vi "G2CPU Complex Process.vi"(10 "Backend":T1 items=["Default Backend"=0, "CPU Backend"=1, "CUDA Backend"=2, "OPENCL Backend"=4, "Intel OneAPI"=8], 11 "X size":i32=16384) -> (3 "G2CPU Time":dbl)   [LabVIEW 2020]
uses:
  <vilib>/Natan Biesmans/G2CPU GPU and CPU HPC Toolkit/ArrayFire Driver/TypeDefs/backend.ctl
  fbbaf97c-3b5e-4b4c-bc14-40c3526c788b.vi
  c2200195-6f6b-46fb-afe8-d4cd0bcb91cf.vi
  fbbaf97c-3b5e-4b4c-bc14-40c3526c788b.vi/caaf1833-0905-411b-a9ed-2cc30d41907c.vi
  <vilib>/Natan Biesmans/G2CPU GPU and CPU HPC Toolkit/G2CPU Libraries/Arrays/SubVI/Array Sizes to Dim Cluster.vi
  c2200195-6f6b-46fb-afe8-d4cd0bcb91cf.vi/caaf1833-0905-411b-a9ed-2cc30d41907c.vi
  fbbaf97c-3b5e-4b4c-bc14-40c3526c788b.vi/caaf1833-0905-411b-a9ed-2cc30d41907c.vi/1a23f98f-393f-4176-8983-7f1ab824c539.vi
  c2200195-6f6b-46fb-afe8-d4cd0bcb91cf.vi/caaf1833-0905-411b-a9ed-2cc30d41907c.vi/1a23f98f-393f-4176-8983-7f1ab824c539.vi
  <vilib>/Natan Biesmans/G2CPU GPU and CPU HPC Toolkit/G2CPU Libraries/Arrays/1DArray/c32/1D Array c32.lvclass
  C:/Program Files/National Instruments/LabVIEW 2020/vi.lib/Natan Biesmans/G2CPU GPU and CPU HPC Toolkit/G2CPU Libraries/Arrays/Array/Array Prototype.lvclass
  <vilib>/Natan Biesmans/G2CPU GPU and CPU HPC Toolkit/G2CPU Libraries/Runtime Licensing/G2CPU License Check.vi
  <vilib>/Natan Biesmans/G2CPU GPU and CPU HPC Toolkit/ArrayFire Driver/VIs/init.vi
  <vilib>/Natan Biesmans/G2CPU GPU and CPU HPC Toolkit/G2CPU Libraries/Async IO/CUDA Context FGV.vi
  <resource>/Natan Biesmans/G2CPU GPU and CPU HPC Toolkit/Garbage Collector/G2CPU GarbageCollectorFGV.vi
  <resource>/Natan Biesmans/G2CPU GPU and CPU HPC Toolkit/Garbage Collector/G2CPU DMAGarbageCollectorFGV.vi
  <vilib>/Natan Biesmans/G2CPU GPU and CPU HPC Toolkit/G2CPU Libraries/Manage Environment/Find AF DLL.vi
  <vilib>/Natan Biesmans/G2CPU GPU and CPU HPC Toolkit/ArrayFire Driver/VIs/Run as Multi Device.vi
  <vilib>/Natan Biesmans/G2CPU GPU and CPU HPC Toolkit/ArrayFire Driver/subvi/Error Converter (ErrCode or Status).vi
  <vilib>/Natan Biesmans/G2CPU GPU and CPU HPC Toolkit/G2CPU Libraries/Arrays/Array/G2CPU Set Array Pointer.vi
  <vilib>/Natan Biesmans/G2CPU GPU and CPU HPC Toolkit/G2CPU Libraries/Arrays/Array/Array Prototype.lvclass
  <vilib>/Natan Biesmans/G2CPU GPU and CPU HPC Toolkit/G2CPU Libraries/Manage Environment/G2CPU Manage Environment.lvlib
  <vilib>/Analysis/NI_AALBase.lvlib
  <vilib>/Natan Biesmans/G2CPU GPU and CPU HPC Toolkit/ArrayFire Driver/AF.lvlib
panel:
  out "Numeric":i32
  out "imag out":dbl
  out "max value":dbl
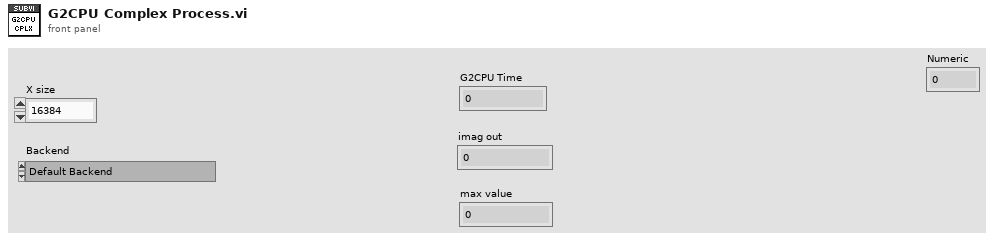
[diagram p1: front panel]
types:
  T1 = typedef "AF.lvlib/backend.ctl" = u32
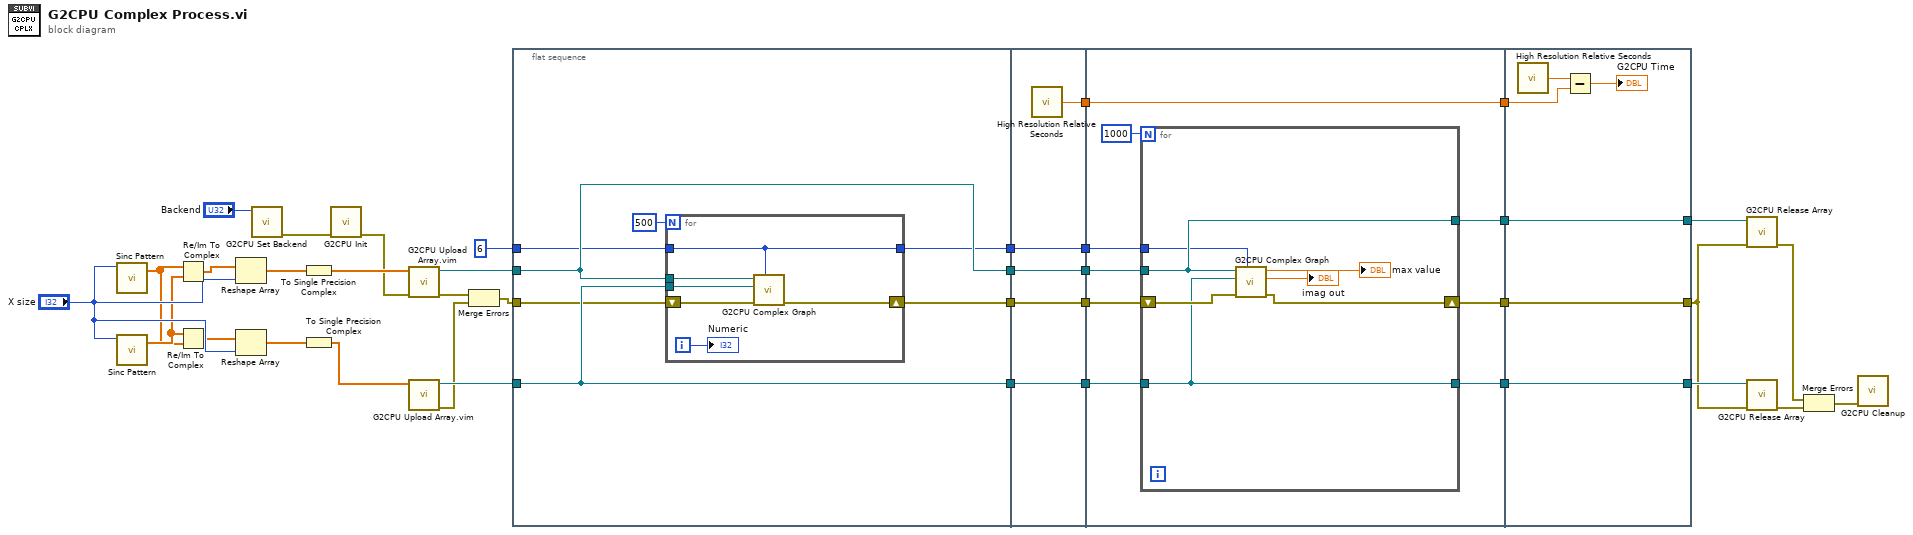
[diagram p0: block diagram]
diagram:
  n1 = call <vilib>:"Sinc Pattern.vi"("samples"="X size") -> ("Sinc Pattern"=w10:dbl[])  [unwired: 3 in, 1 out]
  n2 = call <vilib>:"Sinc Pattern.vi"("samples"="X size") -> ("Sinc Pattern"=w11:dbl[])  [unwired: 3 in, 1 out]
  n3 = Re/Im To Complex(1:w11, 2:w10) -> (0:w12:cdb[])
  n4 = Re/Im To Complex(1:w10, 2:w11) -> (0:w9:cdb[])
  n5 = Reshape Array(w12, "X size") -> (w8:cdb[])
  n6 = Reshape Array(w9, "X size") -> (w7:cdb[])
  n7 = call <vilib>:"G2CPU Set Backend.vi"("Backend"="Backend") -> ("error out"=w17:errorcluster)  [unwired: 10 in]
  n8 = To Single Precision Complex(1:w8) -> (0:w5:csg[])
  n9 = To Single Precision Complex(1:w7) -> (0:w6:csg[])
  n10 = call <vilib>:"G2CPU Init.vi"("error in (no error)"=w17) -> ("error out"=w4:errorcluster)  [unwired: 10 in]
  n11 = call "G2CPU Upload Array.vim"("error in (no error)"=w4, "Data"=w5) -> ("error out"=w28:errorcluster, "Array"=w32:refnum<class "1D Array c32.lvclass">)  [unwired: 8 in]
  n12 = call "G2CPU Upload Array.vim"("Data"=w6) -> ("error out"=w20:errorcluster, "Array"=w31:refnum<class "1D Array c32.lvclass">)  [unwired: 9 in]
  n13 = Merge Errors(w28, w20) -> (w21:errorcluster)
  n14 = flat-sequence {
    tunnel: w32 -> [w40]
    tunnel: [w40] -> w34
    tunnel: w31 -> [w43]
    tunnel: [w43] -> w30
    tunnel: w21 -> [w42]
    tunnel: [w44] -> w26
    tunnel: 6 ("num_loop") -> [w39]
    tunnel: [w38] -> w2
    tunnel: [w55] -> w37
    tunnel: [w54] -> w36
    tunnel: w34 -> [w54]
    tunnel: w30 -> [w53]
    tunnel: [w53] -> w29
    tunnel: [w52] -> w27
    tunnel: w26 -> [w52]
    tunnel: w2 -> [w51]
    tunnel: [w51] -> w1
    tunnel: w37 -> [w64]
    tunnel: [w64] -> w35
    tunnel: w36 -> [w63]
    tunnel: [w61] -> w33
    tunnel: w29 -> [w60]
    tunnel: w27 -> [w59]
    tunnel: [w58] -> w23
    tunnel: [w57] -> w19
    tunnel: w1 -> [w56]
    tunnel: w35 -> [w76]
    tunnel: w33 -> [w74]
    tunnel: [w74] -> w25
    tunnel: [w73] -> w24
    tunnel: w23 -> [w73]
    tunnel: [w72] -> w18
    tunnel: w19 -> [w72]
    frame #0 {
      n15 = for {
        N: 500 -> [_]
        tunnel: w40 -> [w48]
        tunnel: w43 -> [w47]
        shift-right: [w50] -> w44
        shift-left: w42 -> [w49]
        tunnel: w39 -> [w46]
        tunnel: [w46] -> w38
        i -> [w45]
        n16 = call "G2CPU Complex Graph.vi"("num_loop"=w46, "error in (no error)"=w49, "B"=w47, "A"=w48) -> ("error out"=w50:errorcluster)  [unwired: 5 in, 2 out]
        "Numeric" <- w45
      }
    }
    frame #1 {
      n17 = call <vilib>:"High Resolution Relative Seconds.vi"() -> ("relative seconds"=w55:dbl)
    }
    frame #2 {
      n18 = for {
        N: 1000 -> [_]
        tunnel: w63 -> [w68]
        tunnel: [w68] -> w61
        tunnel: w60 -> [w67]
        tunnel: [w67] -> w58
        shift-right: [w69] -> w57
        shift-left: w59 -> [w71]
        tunnel: w56 -> [w66]
        n19 = call "G2CPU Complex Graph.vi"("num_loop"=w66, "error in (no error)"=w71, "B"=w67, "A"=w68) -> ("error out"=w69:errorcluster, "imag out"=→"imag out":dbl, "real out"=→"max value":dbl)  [unwired: 5 in]
      }
    }
    frame #3 {
      n20 = call <vilib>:"High Resolution Relative Seconds.vi"() -> ("relative seconds"=w77:dbl)
      n21 = Subtract(x=w77, y=w76) -> (x-y=→"G2CPU Time":dbl)
    }
  }
  n22 = call <vilib>:"G2CPU Release Array.vi"("error in (no error)"=w18, "Array in"=w25) -> ("error out"=w16:errorcluster)  [unwired: 9 in]
  n23 = call <vilib>:"G2CPU Release Array.vi"("error in (no error)"=w18, "Array in"=w24) -> ("error out"=w14:errorcluster)  [unwired: 9 in]
  n24 = Merge Errors(w16, w14) -> (w15:errorcluster)
  n25 = call <vilib>:"G2CPU Cleanup.vi"("error in (no error)"=w15) -> ()  [unwired: 10 in, 1 out]
